vi "Encoder to Hood.vi"(11 "Encoder":dbl) -> (3 "Hood Angle":dbl)   [LabVIEW 2019]
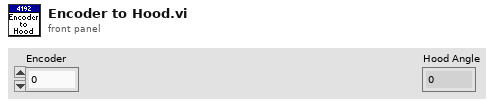
[diagram p1: front panel]
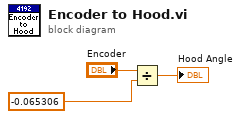
[diagram p0: block diagram]
diagram:
  n1 = Divide(x="Encoder", y=-0.065306) -> (x/y=→"Hood Angle":dbl)
